vi "FastExposureSwitching.vi"() -> ()   [LabVIEW 2009]
uses:
  Data/GetPixelData16.vi
panel:
  out "stop":bool
  in  "NumExposures":dbl
  out "Current Exposure":i32
  in  "Exposure Ring":dbl[](array[numeric])
  out "ExposureEndEvent":refnum<user-event>
  out "Exposure End Refnum":refnum<event-registration>
  in  "NumImages":i32
  in  "Centre AOI":bool
  in  "AOI Width":i64
  in  "AOI Height":i64
  out "Ready":bool
  in  "Run":bool
  in  "error":errorcluster
  out "Pixel Encoding":string
  out "Intensity Graph":u16[][](graph)
  out "AOIStride":i64
  in  "PreAmp":string(combo)
  out "PixelData":u16[](array[numeric])
  out "ByteData":u8[](array[numeric])
  out "ImageSizeBytes":i64
  out "Handle":i32
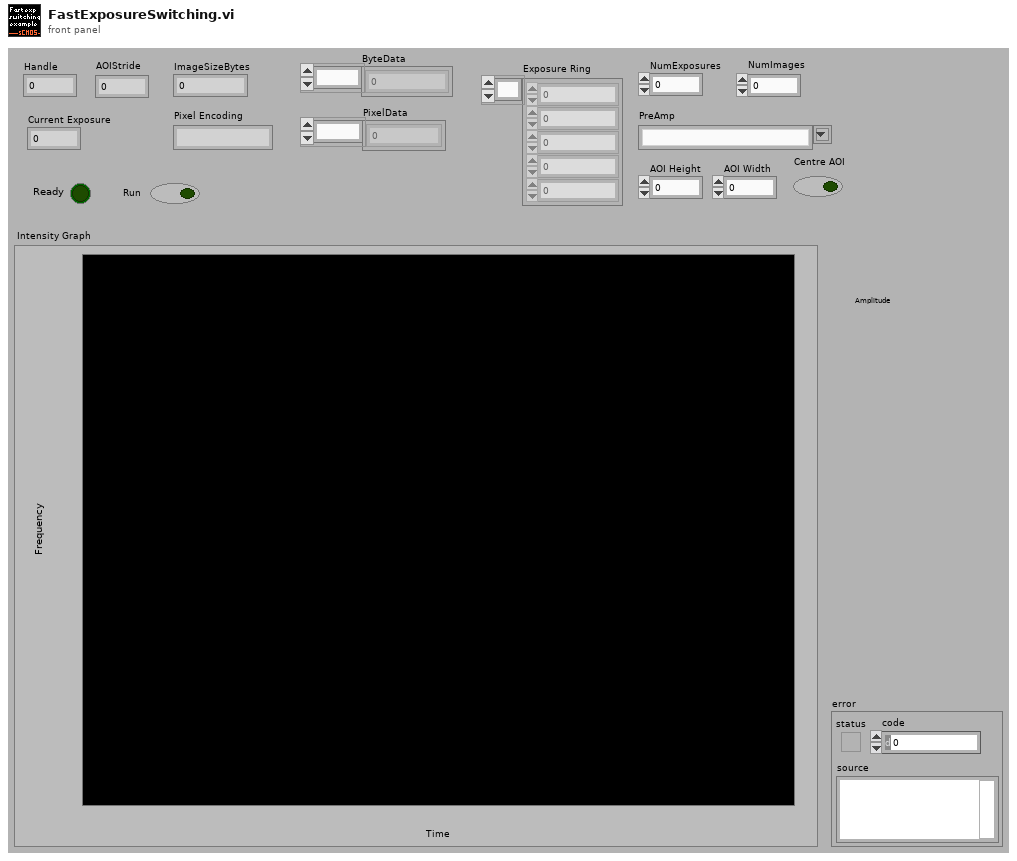
[diagram p1: front panel]
types:
  T1 = enum8{"Enabled", "Disabled", "Disabled and Grayed Out"}
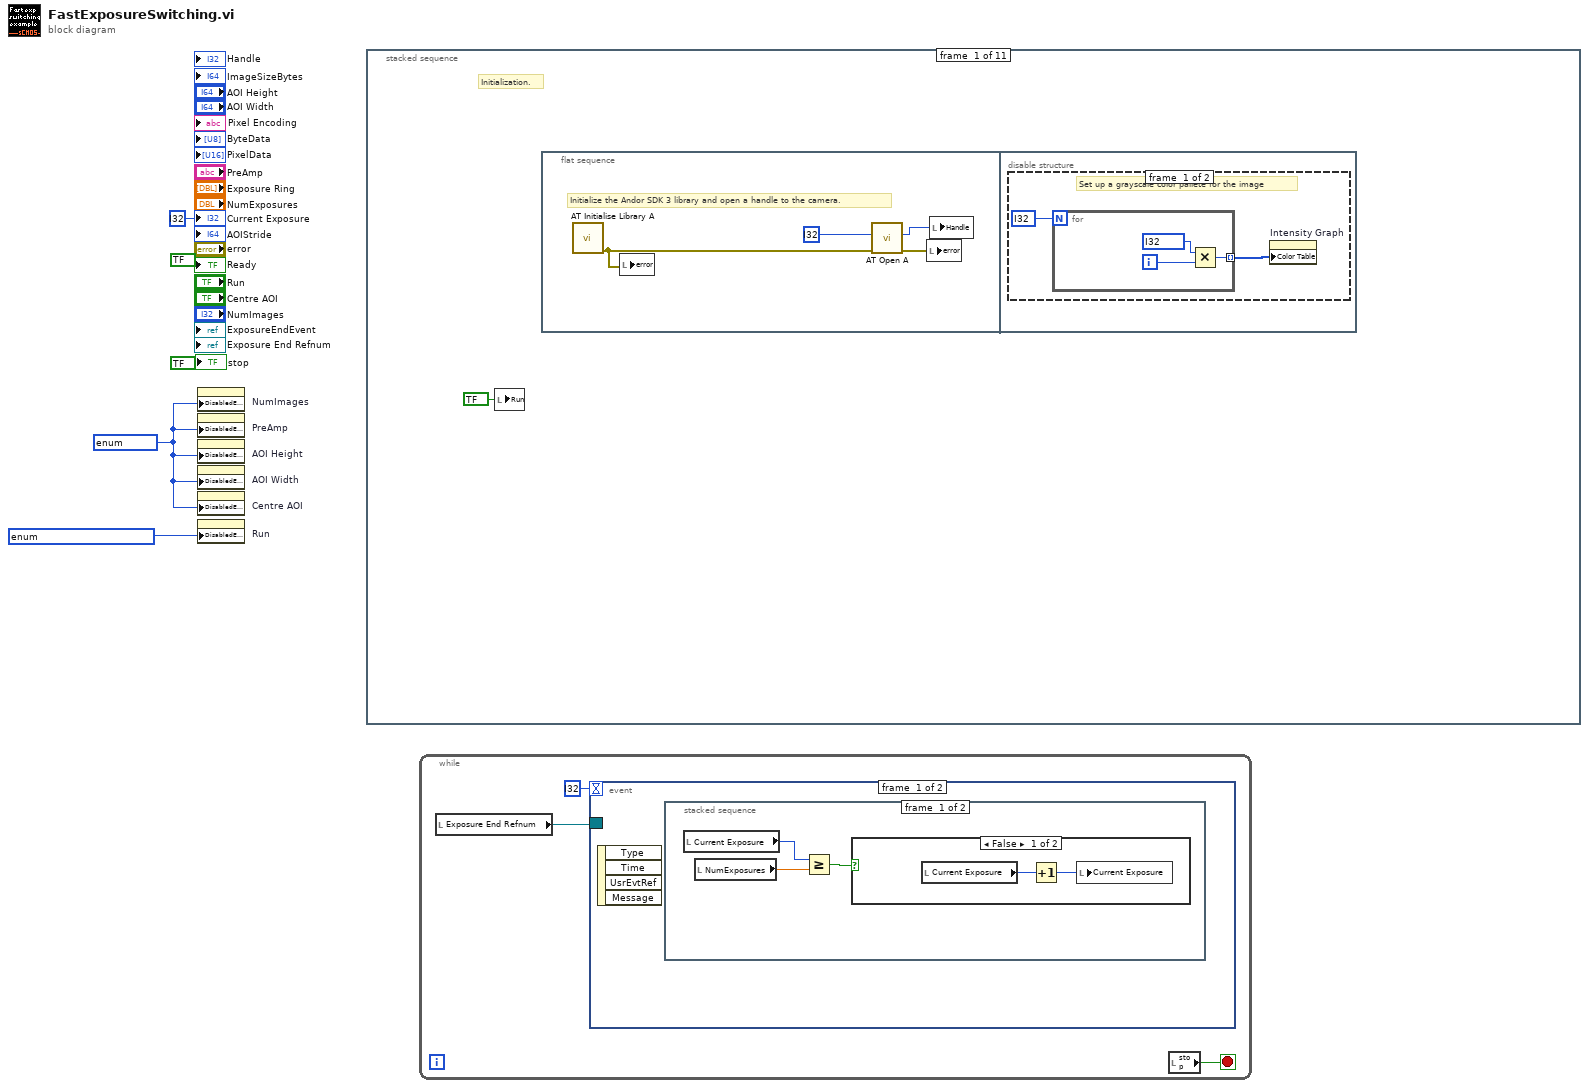
[diagram p0: block diagram]
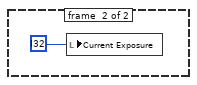
[diagram p2: hidden frame]
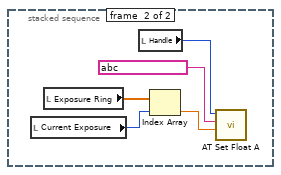
[diagram p3: hidden frame]
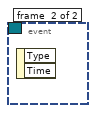
[diagram p4: hidden frame]
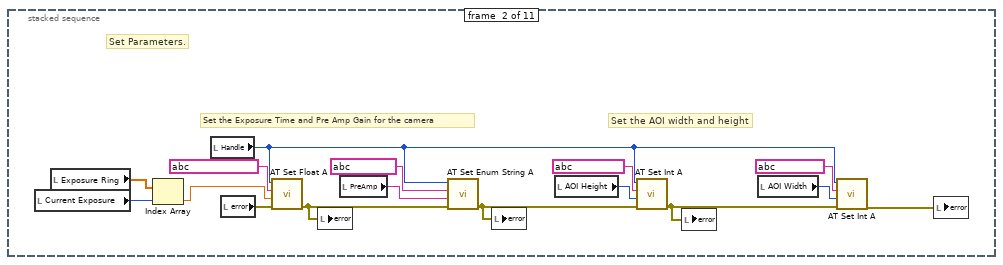
[diagram p6: hidden frame]
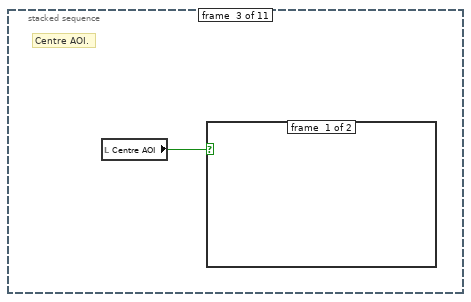
[diagram p7: hidden frame]
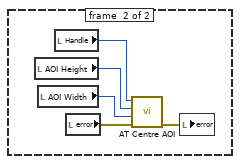
[diagram p8: hidden frame]
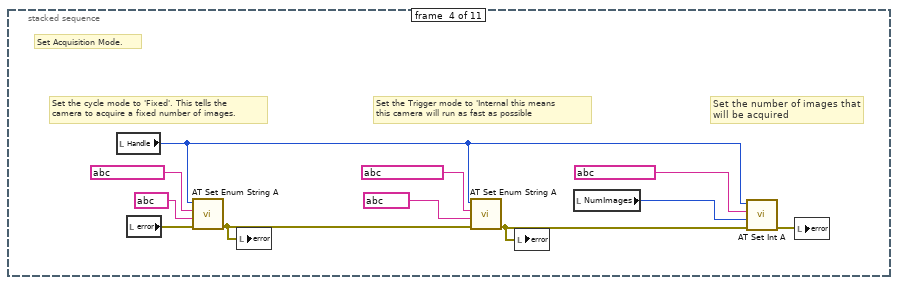
[diagram p9: hidden frame]
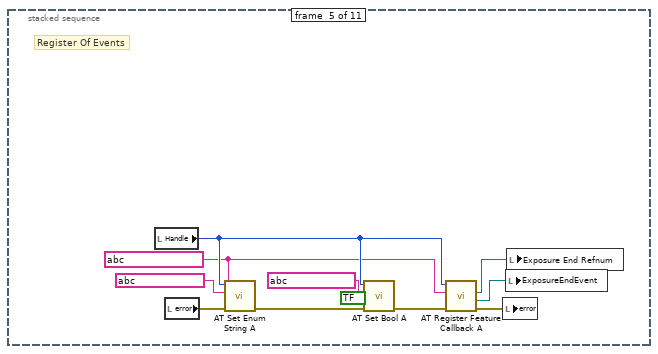
[diagram p10: hidden frame]
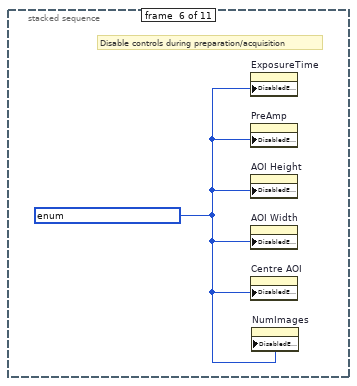
[diagram p11: hidden frame]
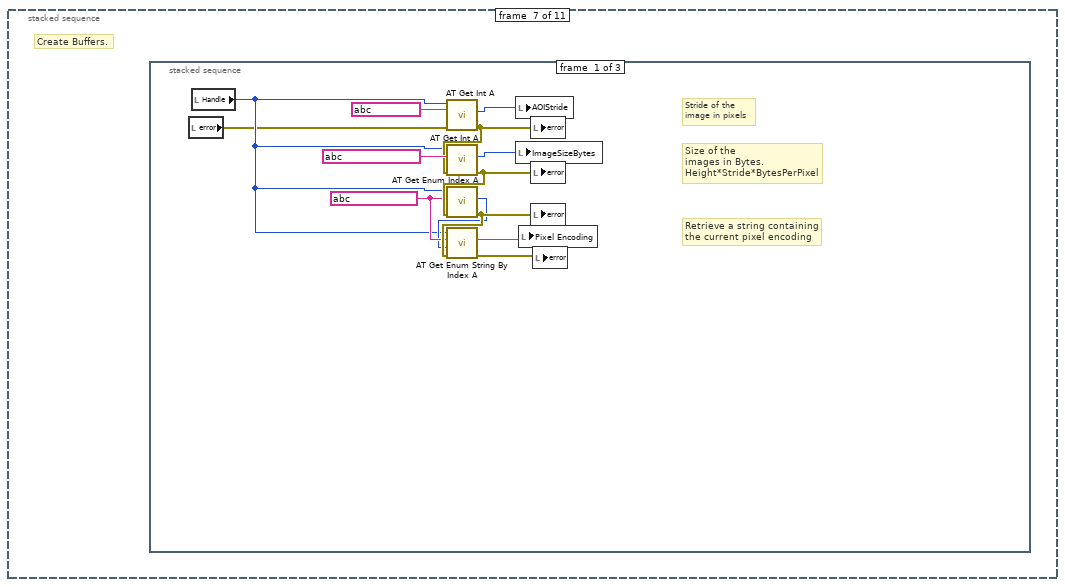
[diagram p12: hidden frame]
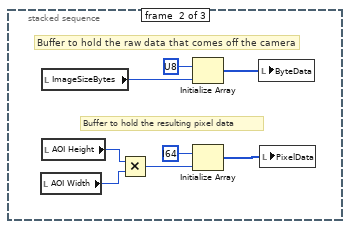
[diagram p13: hidden frame]
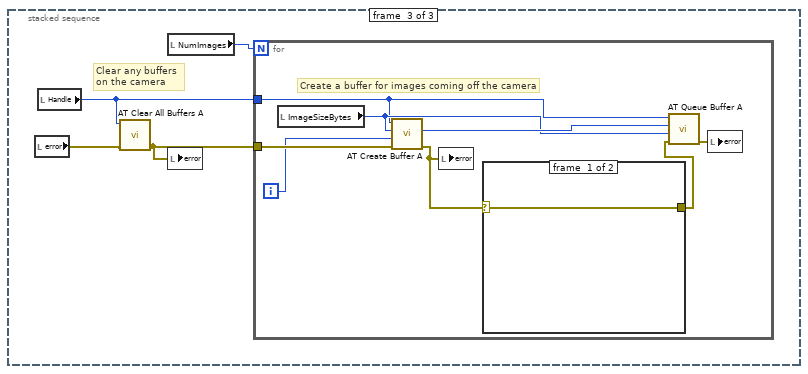
[diagram p14: hidden frame]
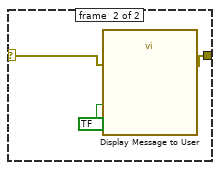
[diagram p15: hidden frame]
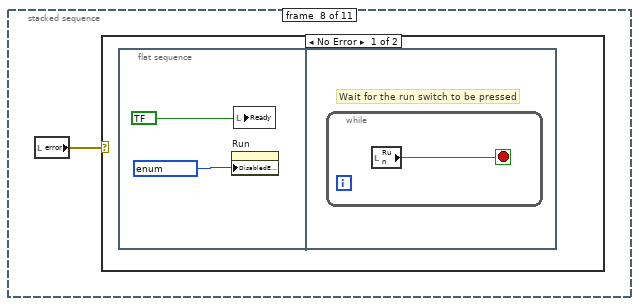
[diagram p16: hidden frame]
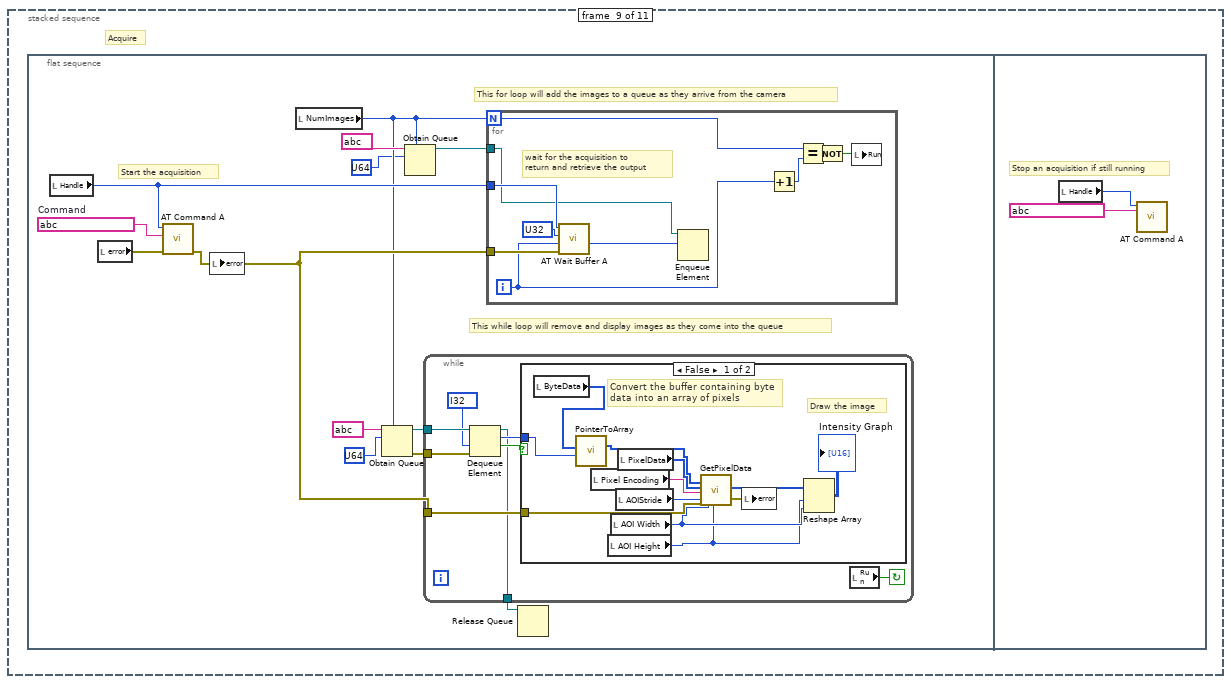
[diagram p18: hidden frame]
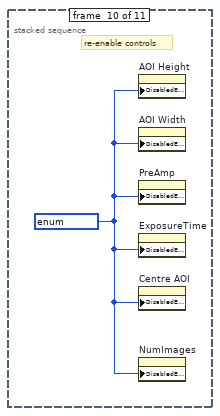
[diagram p20: hidden frame]
diagram:
  w4 = T1 ? ("Disabled")
  n1 = property on="NumImages" class="DigNum (strict)"("DisabledEnum"=w4) -> ()  [unwired: 2 in, 2 out]
  n2 = property on="PreAmp" class="CmbBox"("DisabledEnum"=w4) -> ()  [unwired: 2 in, 2 out]
  n3 = property on="AOI Height" class="DigNum (strict)"("DisabledEnum"=w4) -> ()  [unwired: 2 in, 2 out]
  n4 = property on="AOI Width" class="DigNum (strict)"("DisabledEnum"=w4) -> ()  [unwired: 2 in, 2 out]
  n5 = property on="Centre AOI" class="Bool (strict)"("DisabledEnum"=w4) -> ()  [unwired: 2 in, 2 out]
  n6 = property on="Run" class="Bool (strict)"("DisabledEnum"=T1 ? ("Disabled")) -> ()  [unwired: 2 in, 2 out]
  n7 = stacked-sequence {
    frame #0 {
      # "Initialization."
      n8 = local write "Run"(bool ? ("Run")) -> ()
      n9 = flat-sequence {
        frame #0 {
          # "Initialize the Andor SDK 3 library and open a handle to the camera."
          n10 = call "AT Initialise Library A.vi"() -> ("error out"=w8:errorcluster)  [unwired: 10 in, 1 out]
          n11 = local write "error"(w8) -> ()
          n12 = call "AT Open A.vi"("error in (no error)"=w8, "CameraIndex"=i32 ?) -> ("error out"=w7:errorcluster, "Handle"=w9:i32)  [unwired: 7 in, 1 out]
          n13 = local write "error"(w7) -> ()
          n14 = local write "Handle"(w9) -> ()
        }
        frame #1 {
          n15 = disable-structure shown="Enabled" {
            frame #0 {
              # "Set up a grayscale color pallete for the image"
              n16 = for {
                N: i32 ? -> [_]
                tunnel: [w14] -> w11 mode=indexing
                i -> [w15]
                n17 = Multiply(x=i32 ?, y=w15) -> (x*y=w14:i32)
              }
              n18 = property on="Intensity Graph" class="IntGraph (strict)"("Color Table"=w11) -> ()  [unwired: 2 in, 2 out]
            }
            frame #1 {
            }
          }
        }
      }
    }
    frame #1 {
      # "Set the AOI width and height"
      # "Set the Exposure Time and Pre Amp Gain for the camera"
      # "Set Parameters."
      n19 = local read "Current Exposure"() -> (w18:i32)
      n20 = local read "Exposure Ring"() -> (w17:dbl[])
      n21 = Index Array(array=w17, index=w18) -> (element=w16:dbl)
      n22 = local read "Handle"() -> (w19:i32)
      n23 = local read "error"() -> (w27:errorcluster)
      n24 = call "AT Set Float A.vi"("error in (no error)"=w27, "Value"=w16, "Feature"=string ? ("ExposureTime"), "Hndl"=w19) -> ("error out"=w30:errorcluster)  [unwired: 6 in, 1 out]
      n25 = local write "error"(w30) -> ()
      n26 = local read "PreAmp"() -> (w31:string)
      n27 = call "AT Set Enum String A.vi"("error in (no error)"=w30, "String"=w31, "Feature"=string ? ("SimplePreAmpGainControl"), "Handle"=w19) -> ("error out"=w26:errorcluster)  [unwired: 6 in, 1 out]
      n28 = local write "error"(w26) -> ()
      n29 = local read "AOI Height"() -> (w23:i64)
      n30 = call "AT Set Int A.vi"("error in (no error)"=w26, "Value"=w23, "Feature"=string ? ("Integer feature"), "Handle"=w19) -> ("error out"=w24:errorcluster)  [unwired: 6 in, 1 out]
      n31 = local write "error"(w24) -> ()
      n32 = local read "AOI Width"() -> (w22:i64)
      n33 = call "AT Set Int A.vi"("error in (no error)"=w24, "Value"=w22, "Feature"=string ? ("Integer feature 2"), "Handle"=w19) -> ("error out"=w25:errorcluster)  [unwired: 6 in, 1 out]
      n34 = local write "error"(w25) -> ()
    }
    frame #2 {
      # "Centre AOI."
      n35 = local read "Centre AOI"() -> (w32:bool)
      n36 = case shown="True" w32 {
        frame #0 {
        }
        frame #1 {
          n37 = local read "AOI Height"() -> (w34:i64)
          n38 = local read "AOI Width"() -> (w35:i64)
          n39 = local read "Handle"() -> (w33:i32)
          n40 = local read "error"() -> (w36:errorcluster)
          n41 = call "AT Centre AOI.vi"("error in (no error)"=w36, "AOI Width"=w35, "AOI Height"=w34, "Handle"=w33) -> ("error out"=w37:errorcluster)  [unwired: 7 in]
          n42 = local write "error"(w37) -> ()
        }
      }
    }
    frame #3 {
      # "Set the number of images that \nwill be acquired"
      # "Set the Trigger mode to 'Internal this means \nthis camera will run as fast as possible"
      # "Set the cycle mode to 'Fixed'. This tells the \ncamera to acquire a fixed number of images."
      # "Set Acquisition Mode."
      n43 = local read "Handle"() -> (w39:i32)
      n44 = local read "error"() -> (w46:errorcluster)
      n45 = call "AT Set Enum String A.vi"("error in (no error)"=w46, "String"=string ?, "Feature"=string ? ("Enum feature"), "Handle"=w39) -> ("error out"=w45:errorcluster)  [unwired: 6 in, 1 out]
      n46 = local write "error"(w45) -> ()
      n47 = call "AT Set Enum String A.vi"("error in (no error)"=w45, "String"=string ?, "Feature"=string ? ("Enum feature"), "Handle"=w39) -> ("error out"=w42:errorcluster)  [unwired: 6 in, 1 out]
      n48 = local write "error"(w42) -> ()
      n49 = local read "NumImages"() -> (w40:i32)
      n50 = call "AT Set Int A.vi"("error in (no error)"=w42, "Value"=w40, "Feature"=string ? ("Integer feature 2"), "Handle"=w39) -> ("error out"=w38:errorcluster)  [unwired: 6 in, 1 out]
      n51 = local write "error"(w38) -> ()
    }
    frame #4 {
      w52 = string ? ("String")
      # "Register Of Events"
      n52 = local read "Handle"() -> (w55:i32)
      n53 = local read "error"() -> (w59:errorcluster)
      n54 = call "AT Set Enum String A.vi"("error in (no error)"=w59, "String"=w52, "Feature"=string ? ("Enum feature"), "Handle"=w55) -> ("error out"=w58:errorcluster)  [unwired: 6 in, 1 out]
      n55 = call "AT Set Bool A.vi"("error in (no error)"=w58, "Value"=bool ?, "Feature"=string ? ("Bool feature"), "Handle"=w55) -> ("error out"=w57:errorcluster)  [unwired: 6 in, 1 out]
      n56 = call "AT Register Feature Callback A.vi"("error in (no error)"=w57, "Feature"=w52, "Handle"=w55) -> ("error out"=w51:errorcluster, "Event"=w49:refnum<user-event>, "Event Registration Refnum"=w50:refnum<event-registration>)  [unwired: 5 in, 1 out]
      n57 = local write "error"(w51) -> ()
      n58 = local write "ExposureEndEvent"(w49) -> ()
      n59 = local write "Exposure End Refnum"(w50) -> ()
    }
    frame #5 {
      w60 = T1 ? ("Disabled")
      # "Disable controls during preparation/acquisition"
      n60 = property on="ExposureTime" class="DigNum (strict)"("DisabledEnum"=w60) -> ()  [unwired: 2 in, 2 out]
      n61 = property on="PreAmp" class="CmbBox"("DisabledEnum"=w60) -> ()  [unwired: 2 in, 2 out]
      n62 = property on="AOI Height" class="DigNum (strict)"("DisabledEnum"=w60) -> ()  [unwired: 2 in, 2 out]
      n63 = property on="AOI Width" class="DigNum (strict)"("DisabledEnum"=w60) -> ()  [unwired: 2 in, 2 out]
      n64 = property on="Centre AOI" class="Bool (strict)"("DisabledEnum"=w60) -> ()  [unwired: 2 in, 2 out]
      n65 = property on="NumImages" class="DigNum (strict)"("DisabledEnum"=w60) -> ()  [unwired: 2 in, 2 out]
    }
    frame #6 {
      # "Create Buffers."
      n66 = stacked-sequence {
        frame #0 {
          w66 = string ? ("Enum feature")
          # "Retrieve a string containing \nthe current pixel encoding"
          # "Stride of the\nimage in pixels"
          # "Size of the\nimages in Bytes.\nHeight*Stride*BytesPerPixel"
          n67 = local read "error"() -> (w61:errorcluster)
          n68 = local read "Handle"() -> (w62:i32)
          n69 = call "AT Get Int A.vi"("error in (no error)"=w61, "Feature"=string ? ("Integer feature"), "Handle"=w62) -> ("error out"=w69:errorcluster, "Value"=w73:i64)  [unwired: 6 in, 1 out]
          n70 = call "AT Get Int A.vi"("error in (no error)"=w69, "Feature"=string ? ("Integer feature"), "Handle"=w62) -> ("error out"=w68:errorcluster, "Value"=w72:i64)  [unwired: 6 in, 1 out]
          n71 = call "AT Get Enum Index A.vi"("error in (no error)"=w68, "Feature"=w66, "Handle"=w62) -> ("error out"=w67:errorcluster, "Value"=w65:i32)  [unwired: 6 in, 1 out]
          n72 = call "AT Get Enum String By Index A.vi"("error in (no error)"=w67, "Index"=w65, "Feature"=w66, "Handle"=w62) -> ("error out"=w63:errorcluster, "String"=w64:string)  [unwired: 5 in, 1 out]
          n73 = local write "AOIStride"(w73) -> ()
          n74 = local write "ImageSizeBytes"(w72) -> ()
          n75 = local write "Pixel Encoding"(w64) -> ()
          n76 = local write "error"(w69) -> ()
          n77 = local write "error"(w68) -> ()
          n78 = local write "error"(w67) -> ()
          n79 = local write "error"(w63) -> ()
        }
        frame #1 {
          # "Buffer to hold the resulting pixel data"
          # "Buffer to hold the raw data that comes off the camera"
          n80 = local read "AOI Width"() -> (w80:i64)
          n81 = local read "ImageSizeBytes"() -> (w75:i64)
          n82 = local read "AOI Height"() -> (w79:i64)
          n83 = Multiply(x=w79, y=w80) -> (x*y=w74:i64)
          n84 = Initialize Array(u8 ?, w75) -> (w77:u8[])
          n85 = Initialize Array(i64 ?, w74) -> (w78:i64[])
          n86 = local write "ByteData"(w77) -> ()
          n87 = local write "PixelData"(w78) -> ()
        }
        frame #2 {
          # "Clear any buffers \non the camera"
          n88 = local read "error"() -> (w85:errorcluster)
          n89 = local read "Handle"() -> (w83:i32)
          n90 = call "AT Clear All Buffers A.vi"("error in (no error)"=w85, "Handle"=w83) -> ("error out"=w84:errorcluster)  [unwired: 8 in, 1 out]
          n91 = local read "NumImages"() -> (w82:i32)
          n92 = local write "error"(w84) -> ()
          n93 = for {
            N: w82 -> [_]
            tunnel: w84 -> [w90]
            tunnel: w83 -> [w89]
            i -> [w88]
            # "Create a buffer for images coming off the camera"
            n94 = local read "ImageSizeBytes"() -> (w92:i64)
            n95 = call "AT Create Buffer A.vi"("error in (no error)"=w90, "Buffer"=w88, "Size"=w92, "Handle"=w89) -> ("error out"=w87:errorcluster, "Buffer out"=w93:u64)  [unwired: 5 in, 1 out]
            n96 = local write "error"(w87) -> ()
            n97 = case shown="Error" w87 {
              selector: w87 -> [w94 w97]
              tunnel: [w94 w96] -> w86
              frame #0 {
              }
              frame #1 {
                n98 = call "Display Message to User"("error in (no error)"=w97, "Enable"=bool ?) -> ("error out"=w96:errorcluster)  [unwired: 8 in, 1 out]
              }
            }
            n99 = call "AT Queue Buffer A.vi"("error in (no error)"=w86, "PtrSize"=w92, "Ptr"=w93, "Handle"=w89) -> ("error out"=w91:errorcluster)  [unwired: 6 in, 1 out]
            n100 = local write "error"(w91) -> ()
          }
        }
      }
    }
    frame #7 {
      n101 = local read "error"() -> (w98:errorcluster)
      n102 = case shown="No Error" w98 {
        frame #0 {
          n103 = flat-sequence {
            frame #0 {
              n104 = property on="Run" class="Bool (strict)"("DisabledEnum"=T1 ? ("Disabled")) -> ()  [unwired: 2 in, 2 out]
              n105 = local write "Ready"(bool ? ("Ready")) -> ()
            }
            frame #1 {
              # "Wait for the run switch to be pressed"
              n106 = while {
                stop <- w101 stop-if-true
                n107 = local read "Run"() -> (w101:bool)
              }
            }
          }
        }
        frame #1 {
        }
      }
    }
    frame #8 {
      # "Acquire"
      n108 = flat-sequence {
        frame #0 {
          w112 = string ?  # Command
          # "This while loop will remove and display images as they come into the queue"
          # "This for loop will add the images to a queue as they arrive from the camera"
          # "Start the acquisition"
          n109 = local read "Handle"() -> (w114:i32)
          n110 = local read "error"() -> (w113:errorcluster)
          n111 = call "AT Command A.vi"("error in (no error)"=w113, "Feature"=w112, "Handle"=w114) -> ("error out"=w111:errorcluster)  [unwired: 7 in, 1 out]
          n112 = local write "error"(w111) -> ()
          n113 = local read "NumImages"() -> (w107:i32)
          n114 = Obtain Queue(max queue size (-1, unlimited)=w107, name (unnamed)=string ?, element data type=u64 ?) -> (queue out=w105:refnum<queue>, error out=w106:errorcluster)  [unwired: 2 in, 1 out]
          n115 = Obtain Queue(max queue size (-1, unlimited)=w107, name (unnamed)=string ?, element data type=u64 ?) -> (queue out=w109:refnum<queue>)  [unwired: 2 in, 2 out]
          n116 = while {
            tunnel: w106 -> [w122]
            tunnel: w105 -> [w121]
            tunnel: w111 -> [w119]
            tunnel: [w115] -> w102
            stop <- w120 continue-if-true
            n117 = Dequeue Element(queue=w121, timeout in ms (-1)=i32 ?, error in (no error)=w122) -> (queue out=w115:refnum<queue>, element=w117:u64, timed out?=w116:bool)  [unwired: 1 out]
            n118 = case shown="False" w116 {
              tunnel: w119 -> [w128 _]
              tunnel: w117 -> [w124 _]
              frame #0 {
                # "Draw the image"
                # "Convert the buffer containing byte \ndata into an array of pixels"
                n119 = local read "ByteData"() -> (w125:u8[])
                n120 = call "PointerToArray.vi"("Pointer In"=w124, "Array in"=w125) -> ("Array out"=w126:u8[])  [unwired: 8 in, 1 out]
                n121 = local read "Pixel Encoding"() -> (w133:string)
                n122 = local read "AOI Height"() -> (w123:i64)
                n123 = local read "AOI Width"() -> (w127:i64)
                n124 = local read "AOIStride"() -> (w134:i64)
                n125 = local read "PixelData"() -> (w132:u16[])
                n126 = call-poly "GetPixelData.vi"("Input buffer"=w126, "Output buffer in"=w132, "Pixel Encoding"=w133, "Stride"=w134, "error in (no error)"=w128, "Width"=w127, "Height"=w123) -> ("Output buffer out"=w129:u16[], "error out"=w131:errorcluster)  [unwired: 10 in, 1 out]
                n127 = local write "error"(w131) -> ()
                n128 = Reshape Array(w129, w123, w127) -> (→"Intensity Graph":u16[][])
              }
              frame #1 {
              }
            }
            n129 = local read "Run"() -> (w120:bool)
          }
          n130 = for {
            N: w107 -> [w139]
            tunnel: w114 -> [w143]
            tunnel: w111 -> [w142]
            tunnel: w109 -> [w141]
            i -> [w138]
            # "wait for the acquisition to \nreturn and retrieve the output"
            n131 = call "AT Wait Buffer A.vi"("error in (no error)"=w142, "Input buffer"=w138, "Timeout"=u32 ?, "Handle"=w143) -> ("Output buffer"=w140:u64)  [unwired: 4 in, 3 out]
            n132 = Enqueue Element(queue=w141, element=w140) -> ()  [unwired: 2 in, 3 out]
            n133 = Increment(x=w138) -> (x+1=w135:i32)
            n134 = Equal?(x=w139, y=w135) -> (x = y?=w137:bool)
            n135 = Not(x=w137) -> (.not. x?=w136:bool)
            n136 = local write "Run"(w136) -> ()
          }
          n137 = Release Queue(queue=w102) -> ()  [unwired: 2 in, 3 out]
        }
        frame #1 {
          # "Stop an acquisition if still running"
          n138 = local read "Handle"() -> (w146:i32)
          n139 = call "AT Command A.vi"("Feature"=string ? ("Command"), "Handle"=w146) -> ()  [unwired: 8 in, 2 out]
        }
      }
    }
    frame #9 {
      w147 = T1 ? ("Disabled")
      # "re-enable controls"
      n140 = property on="AOI Height" class="DigNum (strict)"("DisabledEnum"=w147) -> ()  [unwired: 2 in, 2 out]
      n141 = property on="AOI Width" class="DigNum (strict)"("DisabledEnum"=w147) -> ()  [unwired: 2 in, 2 out]
      n142 = property on="PreAmp" class="CmbBox"("DisabledEnum"=w147) -> ()  [unwired: 2 in, 2 out]
      n143 = property on="ExposureTime" class="DigNum (strict)"("DisabledEnum"=w147) -> ()  [unwired: 2 in, 2 out]
      n144 = property on="Centre AOI" class="Bool (strict)"("DisabledEnum"=w147) -> ()  [unwired: 2 in, 2 out]
      n145 = property on="NumImages" class="DigNum (strict)"("DisabledEnum"=w147) -> ()  [unwired: 2 in, 2 out]
    }
    frame #10 {
      # "Close the current camera handle and unload the library"
      # "ShutDown."
      n146 = local write "Ready"(bool ? ("Ready")) -> ()
      n147 = local write "stop"(bool ?) -> ()
      n148 = local read "Handle"() -> (w150:i32)
      n149 = call "AT Clear All Buffers A.vi"("Handle"=w150) -> ("error out"=w149:errorcluster)  [unwired: 9 in, 1 out]
      n150 = call "AT Close A.vi"("error in (no error)"=w149, "Handle"=w150) -> ("error out"=w151:errorcluster)  [unwired: 8 in, 1 out]
      n151 = call "AT Finalise Library A.vi"("error in (no error)"=w151) -> ()  [unwired: 9 in, 2 out]
    }
  }
  n152 = while {
    stop <- w153 stop-if-true
    n153 = local read "Exposure End Refnum"() -> (w155:refnum<event-registration>)
    n154 = event shown="[1] Timeout" {
      selector: w155 -> [_ _]
      dyn-events: _ -> [_ _]
      timeout: i32 ? -> [_ _]
      event #0 {
        n155 = event-data() -> ()  [unwired: 1 in, 4 out]
        n156 = stacked-sequence {
          frame #0 {
            n157 = local read "Current Exposure"() -> (w158:i32)
            n158 = local read "NumExposures"() -> (w157:dbl)
            n159 = Greater Or Equal?(x=w158, y=w157) -> (x >= y?=w156:bool)
            n160 = case shown="False" w156 {
              frame #0 {
                n161 = local read "Current Exposure"() -> (w160:i32)
                n162 = Increment(x=w160) -> (x+1=w159:i32)
                n163 = local write "Current Exposure"(w159) -> ()
              }
              frame #1 {
                n164 = local write "Current Exposure"(i32 ? ("Current Exposure")) -> ()
              }
            }
          }
          frame #1 {
            n165 = local read "Current Exposure"() -> (w162:i32)
            n166 = local read "Exposure Ring"() -> (w163:dbl[])
            n167 = local read "Handle"() -> (w166:i32)
            n168 = Index Array(array=w163, index=w162) -> (element=w164:dbl)
            n169 = call "AT Set Float A.vi"("Value"=w164, "Feature"=string ? ("ExposureTime"), "Hndl"=w166) -> ()  [unwired: 7 in, 2 out]
          }
        }
      }
      event #1 {
        n170 = event-data() -> ()  [unwired: 1 in, 2 out]
      }
    }
    n171 = local read "stop"() -> (w153:bool)
  }
  "Ready" <- bool ? ("Ready")
  "Current Exposure" <- i32 ? ("Current Exposure")
  "stop" <- bool ? ("stop")
